vi "No request remaining.vi"(8 "error in (no error)":errorcluster, 11 "Elevator Controller Actor in":refnum<class "Elevator Controller Actor.lvclass">) -> (0 "error out":errorcluster, 3 "Elevator Controller Actor out":refnum<class "Elevator Controller Actor.lvclass">)   [LabVIEW 2019, in "Elevator Controller Actor.lvlib" / "Elevator Controller Actor.lvclass"]
uses:
  Elevator Controller Actor.lvclass
  Sim Display Console Actor/Sim Display Console Actor Messages/Write Timing Msg/Write Timing Msg.lvclass
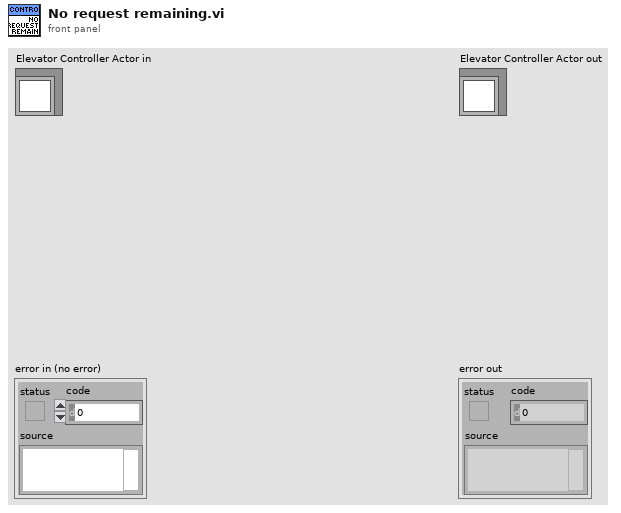
[diagram p1: front panel]
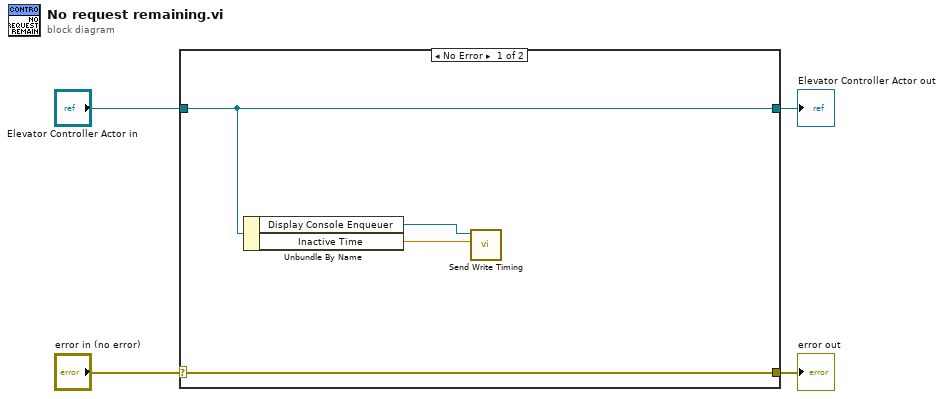
[diagram p0: block diagram]
diagram:
  n1 = case shown="No Error" "error in (no error)" {
    selector: "error in (no error)" -> [w8 w10]
    tunnel: [w8 w10] -> w3
    tunnel: [w6 w9] -> w1
    tunnel: "Elevator Controller Actor in" -> [w6 w9]
    frame No Error {
      n2 = Unbundle By Name(w6) -> ("Display Console Enqueuer"=w5:refnum<class "Message Enqueuer.lvclass">, "Inactive Time"=w7:dbl)
      n3 = call "Send Write Timing.vi"("Time"=w7, "Message Enqueuer"=w5) -> ()  [unwired: 8 in, 2 out]
    }
    frame Error {
    }
  }
  "error out" <- w3
  "Elevator Controller Actor out" <- w1
